vi "Degrees to rad.vi"(10 "Angle array Degrees":dbl[](array[numeric])) -> (2 "Angle array Radians":dbl[](array[numeric]))   [LabVIEW 2015]
doc: "This VI converts all the angles from degrees to radians."
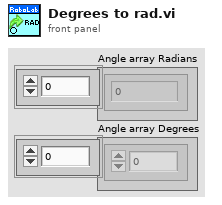
[diagram p1: front panel]
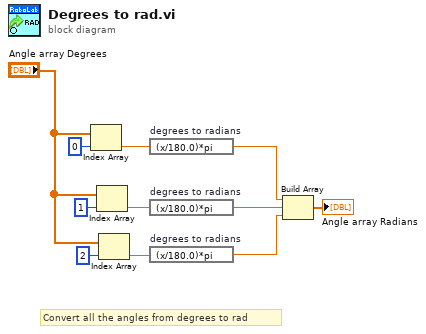
[diagram p0: block diagram]
diagram:
  # "Convert all the angles from degrees to rad"
  n1 = Index Array(array="Angle array Degrees", index=0) -> (element=w5:dbl)
  n2 = Index Array(array="Angle array Degrees", index=1) -> (element=w7:dbl)
  n3 = Index Array(array="Angle array Degrees", index=2) -> (element=w6:dbl)
  n4 = expression code="(x/180.0)*pi" "degrees to radians"(w5) -> (w3:dbl)
  n5 = expression code="(x/180.0)*pi" "degrees to radians"(w7) -> (w1:dbl)
  n6 = expression code="(x/180.0)*pi" "degrees to radians"(w6) -> (w2:dbl)
  n7 = Build Array(w3, w1, w2) -> (→"Angle array Radians":dbl[])
